vi "query_cmd.vi"(6 "Number of bytes in response":u32, 8 "error in (no error)":errorcluster, 9 "Data bytes":u8[](array[numeric]) format="%x", 10 "Command byte":u8=1 format="%x", 11 "VISA resource name":refnum<visa-resource-name>) -> (0 "error out":errorcluster, 2 "Response":string, 3 "VISA resource name out":refnum<visa-resource-name>)   [LabVIEW 2018]
panel:
  out "return count":u32
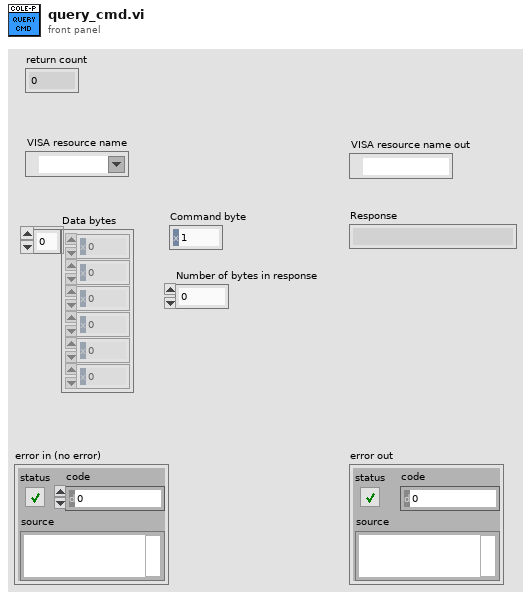
[diagram p1: front panel]
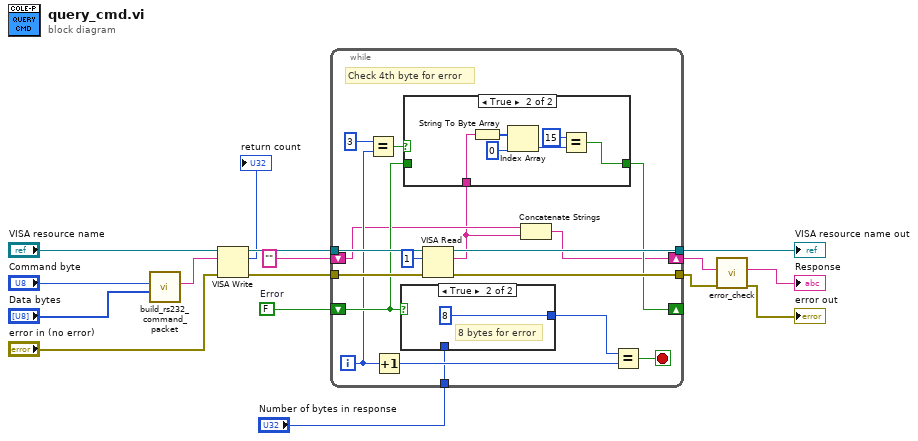
[diagram p0: block diagram]
diagram:
  w3 = FALSE  # Error
  n1 = call "build_rs232_command_packet.vi"("Data bytes"="Data bytes", "Command byte"="Command byte") -> ("Command packet"=w12:string)  [unwired: 9 in]
  n2 = VISA Write(VISA resource name="VISA resource name", write buffer=w12, error in (no error)="error in (no error)") -> (VISA resource name out=w11:refnum<visa-resource-name>, return count=→"return count":u32, error out=w10:errorcluster)
  n3 = while {
    tunnel: "Number of bytes in response" -> [w25]
    shift-right: [w23] -> _
    shift-left: w3 -> [w24]
    shift-right: [w17] -> w8
    shift-left: "" ("read buffer") -> [w19]
    tunnel: w10 -> [w32]
    tunnel: [w30] -> w7
    tunnel: w11 -> [w33]
    tunnel: [w31] -> w9
    i -> [w21]
    stop <- w27 stop-if-true
    # "Check 4th byte for error"
    n4 = Equal?(x=3, y=w21) -> (x = y?=w22:bool)
    n5 = Increment(x=w21) -> (x+1=w28:i32)
    n6 = case shown="True" w24 {
      tunnel: [w41 8] -> w26
      tunnel: w25 -> [w41 _]
      frame False {
      }
      frame True {
        # "8 bytes for error"
      }
    }
    n7 = VISA Read(VISA resource name=w33, byte count=u32 1, error in (no error)=w32) -> (VISA resource name out=w31:refnum<visa-resource-name>, read buffer=w18:string, error out=w30:errorcluster)  [unwired: 1 out]
    n8 = case shown="True" w22 {
      tunnel: w24 -> [w34 _]
      tunnel: [w34 w35] -> w23
      tunnel: w18 -> [_ w37]
      frame False {
      }
      frame True {
        n9 = String To Byte Array(string=w37) -> (unsigned byte array=w40:u8[])
        n10 = Index Array(array=w40, index=0) -> (element=w39:u8)
        n11 = Equal?(x=u8 15, y=w39) -> (x = y?=w35:bool)
      }
    }
    n12 = Concatenate Strings(w19, w18) -> (w17:string)
    n13 = Equal?(x=w26, y=w28) -> (x = y?=w27:bool)
  }
  "VISA resource name out" <- w9
  n14 = call "error_check.vi"("error in (no error)"=w7, "Response in"=w8) -> ("error out"=→"error out":errorcluster, "Response out"=→"Response":string)  [unwired: 8 in]
